vi "MX100 Filter Data.vi"(6 "Base Time":i32, 8 "error in (no error)":errorcluster, 10 "Measurement Values in":dbl[][](array[numeric]), 11 "Measurement Date Times":T2(array[cluster])) -> (0 "error out":errorcluster, 3 "MX100 Data":T1)   [LabVIEW 2016]
uses:
  Type Definitions/MX100 Data.ctl
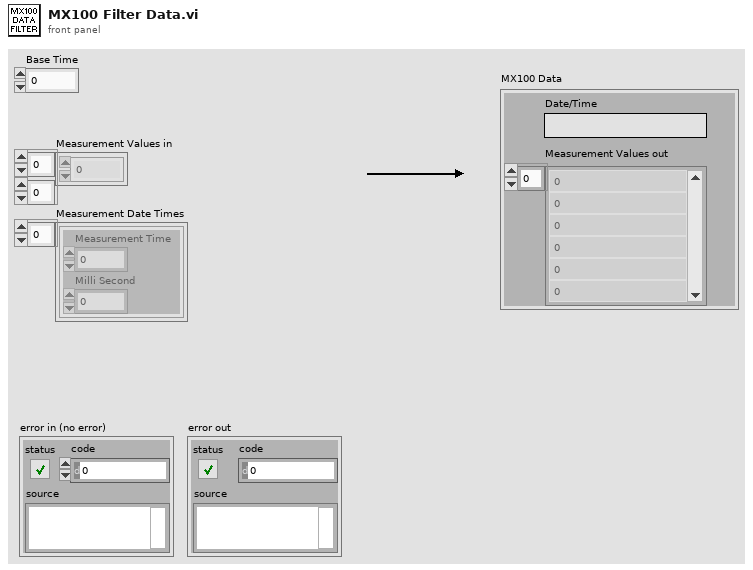
[diagram p1: front panel]
types:
  T1 = typedef "MX100 Data.ctl" = cluster{"Measurement Values out":dbl[], "Date/Time":string}
  T2 = cluster{"Measurement Time":u32, "Milli Second":i32}[]
  T3 = cluster{"Measurement Time":u32, "Milli Second":i32}
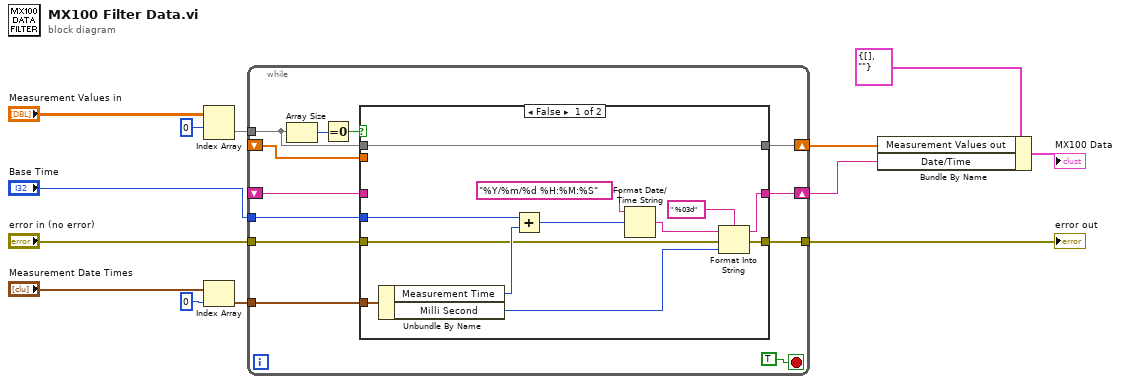
[diagram p0: block diagram]
diagram:
  n1 = Index Array(array="Measurement Values in", index (row)=0) -> (element=w7:dbl[])  [unwired: 1 in]
  n2 = Index Array(array="Measurement Date Times", index=0 ("index (row)")) -> (element=w11:T3)
  n3 = while {
    tunnel: w7 -> [w22]
    shift-right: [w21] -> w3
    shift-left: _ -> [w20]
    tunnel: "Base Time" -> [w14]
    tunnel: w11 -> [w19]
    tunnel: "error in (no error)" -> [w18]
    tunnel: [w17] -> w13
    shift-right: [w16] -> w2
    shift-left: _ -> [w15]
    stop <- TRUE stop-if-true
    n4 = Array Size(array=w22) -> (size(s)=w23:i32)
    n5 = Equal To 0?(x=w23) -> (x = 0?=w24:bool)
    n6 = case shown="False" w24 {
      tunnel: w22 -> [w37 _]
      tunnel: [w37 w40] -> w21
      tunnel: w20 -> [_ w40]
      tunnel: w19 -> [w30 _]
      tunnel: w18 -> [w29 w39]
      tunnel: [w28 w39] -> w17
      tunnel: [w27 w38] -> w16
      tunnel: w15 -> [_ w38]
      tunnel: w14 -> [w26 _]
      frame False {
        n7 = Unbundle By Name(w30) -> ("Measurement Time"=w35:u32, "Milli Second"=w36:i32)
        n8 = Add(x=w26, y=w35) -> (x+y=w32:u32)
        n9 = Format Date/Time String(time format string (%c)="%Y/%m/%d %H:%M:%S", seconds (now)=w32) -> (date/time string=w34:string)  [unwired: 1 in]
        n10 = Format Into String(format string=" %03d", initial string=w34, error in=w29, w36) -> (resulting string=w27:string, error out=w28:errorcluster)
      }
      frame True {
      }
    }
  }
  "error out" <- w13
  n11 = Bundle By Name(cluster=T1 {"Measurement Values out"=[], "Date/Time"=""} ("MX100 Data"), "Measurement Values out"=w3, "Date/Time"=w2) -> (→"MX100 Data":T1)
